vi "ke37xx Channel Pattern.vi"(0 "VISA Resource Name":refnum<visa-resource-name>, 1 "Channel List":string, 5 "Name":string, 7 "Operation (0: Create)":T1(ring), 11 "error in (no error)":errorcluster, 12 "Bytes To Read (1024)":u32=1024) -> (4 "VISA Resource Name Out":refnum<visa-resource-name>, 8 "Pattern Channels":string, 15 "error out":errorcluster)   [LabVIEW 2009, in "Keithley 3700 Series.lvlib"]
doc: "This VI allows you to create, delete, or query a channel pattern. The items specified in the Channel List parameter are associated with the specified Pattern Name."
uses:
  <instrlib>/Keithley 3706/Keithley 3700 Series.lvlib
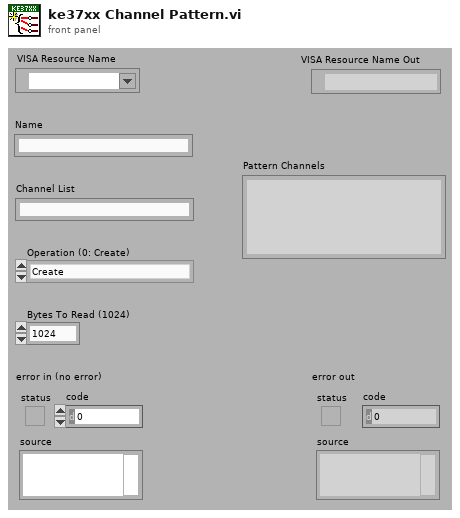
[diagram p1: front panel]
types:
  T1 = enum16{"Create", "Create Snapshot", "Delete", "Query"}
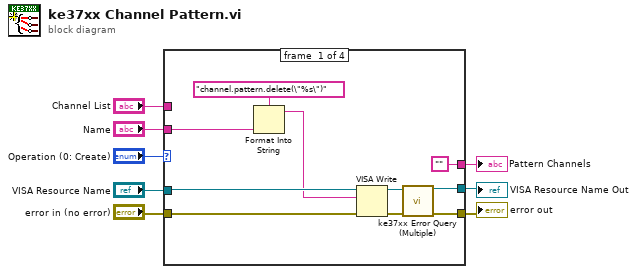
[diagram p0: block diagram]
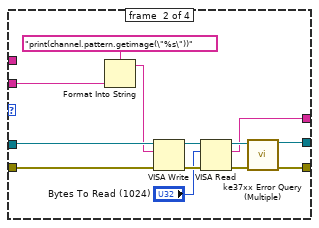
[diagram p2: hidden frame]
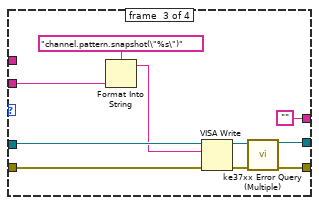
[diagram p3: hidden frame]
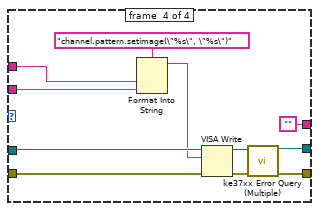
[diagram p4: hidden frame]
diagram:
  n1 = case shown="\"Create Snapshot\"" "Operation (0: Create)" {
    tunnel: "VISA Resource Name" -> [w14 w29 w37 w48]
    tunnel: "error in (no error)" -> [w13 w28 w36 w47]
    tunnel: [w16 w31 w39 w50] -> w6
    tunnel: [w15 w30 w38 w49] -> w5
    tunnel: "Name" -> [w11 w26 w34 w44]
    tunnel: ["" w20 "" ""] -> w2
    tunnel: "Channel List" -> [_ _ _ w42]
    frame #0 {
      n2 = Format Into String(format string="channel.pattern.delete(\"%s\")", w11) -> (resulting string=w10:string)  [unwired: 2 in, 1 out]
      n3 = VISA Write(VISA resource name=w14, write buffer=w10, error in (no error)=w13) -> (VISA resource name out=w18:refnum<visa-resource-name>, error out=w17:errorcluster)  [unwired: 1 out]
      n4 = call <instrlib>:"ke37xx Error Query (Multiple).vi"("VISA resource name"=w18, "error in (no error)"=w17) -> ("VISA resource name out"=w16:refnum<visa-resource-name>, "error out"=w15:errorcluster)  [unwired: 12 out]
    }
    frame #1 {
      n5 = Format Into String(format string="print(channel.pattern.getimage(\"%s\"))", w26) -> (resulting string=w25:string)  [unwired: 2 in, 1 out]
      n6 = VISA Write(VISA resource name=w29, write buffer=w25, error in (no error)=w28) -> (VISA resource name out=w24:refnum<visa-resource-name>, error out=w22:errorcluster)  [unwired: 1 out]
      n7 = VISA Read(VISA resource name=w24, byte count="Bytes To Read (1024)", error in (no error)=w22) -> (VISA resource name out=w23:refnum<visa-resource-name>, read buffer=w20:string, error out=w21:errorcluster)  [unwired: 1 out]
      n8 = call <instrlib>:"ke37xx Error Query (Multiple).vi"("VISA resource name"=w23, "error in (no error)"=w21) -> ("VISA resource name out"=w31:refnum<visa-resource-name>, "error out"=w30:errorcluster)  [unwired: 12 out]
    }
    frame #2 {
      n9 = Format Into String(format string="channel.pattern.snapshot(\"%s\")", w34) -> (resulting string=w33:string)  [unwired: 2 in, 1 out]
      n10 = VISA Write(VISA resource name=w37, write buffer=w33, error in (no error)=w36) -> (VISA resource name out=w41:refnum<visa-resource-name>, error out=w40:errorcluster)  [unwired: 1 out]
      n11 = call <instrlib>:"ke37xx Error Query (Multiple).vi"("VISA resource name"=w41, "error in (no error)"=w40) -> ("VISA resource name out"=w39:refnum<visa-resource-name>, "error out"=w38:errorcluster)  [unwired: 12 out]
    }
    frame #3 {
      n12 = Format Into String(format string="channel.pattern.setimage(\"%s\", \"%s\")", w42, w44) -> (resulting string=w45:string)  [unwired: 2 in, 1 out]
      n13 = VISA Write(VISA resource name=w48, write buffer=w45, error in (no error)=w47) -> (VISA resource name out=w52:refnum<visa-resource-name>, error out=w51:errorcluster)  [unwired: 1 out]
      n14 = call <instrlib>:"ke37xx Error Query (Multiple).vi"("VISA resource name"=w52, "error in (no error)"=w51) -> ("VISA resource name out"=w50:refnum<visa-resource-name>, "error out"=w49:errorcluster)  [unwired: 12 out]
    }
  }
  "VISA Resource Name Out" <- w6
  "error out" <- w5
  "Pattern Channels" <- w2
